vi "Array_to_Spreadsheet.vi"(1 "Headers":string[](array[string]), 2 "Input Array":dbl[][](array[numeric])) -> (0 "spreadsheet string":string)   [LabVIEW 2015]
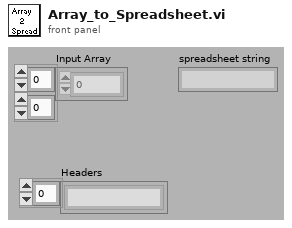
[diagram p1: front panel]
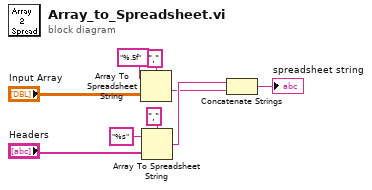
[diagram p0: block diagram]
diagram:
  n1 = Array To Spreadsheet String(delimiter (Tab)=",", array="Input Array", 3:"%.5f" ("format string")) -> (spreadsheet string=w1:string)
  n2 = Array To Spreadsheet String(delimiter (Tab)=",", array="Headers", 3:"%s" ("format string")) -> (spreadsheet string=w3:string)
  n3 = Concatenate Strings(w3, w1) -> (→"spreadsheet string":string)
